vi "p11y3.vi"() -> ()   [LabVIEW 2020]
panel:
  in  "Tegevus 2":enum16{"lahuta", "liida", "alg", "loe"}(ring)
  in  "Tegevus":enum16{"lahuta", "liida", "alg", "loe"}(ring)=enum."liida"
  out "v22rtus":dbl
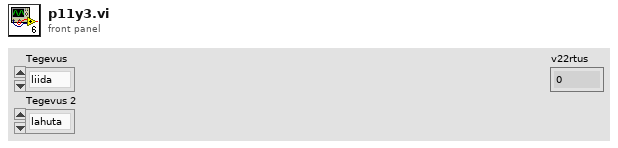
[diagram p1: front panel]
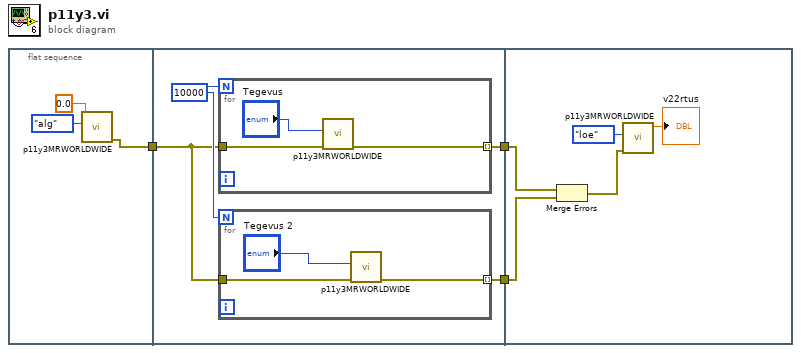
[diagram p0: block diagram]
diagram:
  n1 = flat-sequence {
    tunnel: [w4] -> w3
    tunnel: w3 -> [w9]
    tunnel: [w8] -> w2
    tunnel: [w7] -> w1
    tunnel: w2 -> [w19]
    tunnel: w1 -> [w18]
    frame #0 {
      n2 = call "p11y3MRWORLDWIDE.vi"("Tegevus"=enum16{"lahuta", "liida", "alg", "loe"}."alg", "algv22rtus"=0.0) -> ("error out"=w4:errorcluster)  [unwired: 8 in, 1 out]
    }
    frame #1 {
      w10 = 10000
      n3 = for {
        N: w10 -> [_]
        tunnel: w9 -> [w15]
        tunnel: [w14] -> w8 mode=indexing
        n4 = call "p11y3MRWORLDWIDE.vi"("error in (no error)"=w15, "Tegevus"="Tegevus") -> ("error out"=w14:errorcluster)  [unwired: 8 in, 1 out]
      }
      n5 = for {
        N: w10 -> [_]
        tunnel: w9 -> [w12]
        tunnel: [w11] -> w7 mode=indexing
        n6 = call "p11y3MRWORLDWIDE.vi"("error in (no error)"=w12, "Tegevus"="Tegevus 2") -> ("error out"=w11:errorcluster)  [unwired: 8 in, 1 out]
      }
    }
    frame #2 {
      n7 = Merge Errors(w19, w18) -> (w17:errorcluster)
      n8 = call "p11y3MRWORLDWIDE.vi"("error in (no error)"=w17, "Tegevus"=enum16{"lahuta", "liida", "alg", "loe"}."loe") -> ("v22rtus"=→"v22rtus":dbl)  [unwired: 8 in, 1 out]
    }
  }
